vi "Lab Panel V4.90.vi"() -> ()   [LabVIEW 2013] (continued)
                            n2187 = Build Array(w4046) -> (w4034:dbl[])
                            n2188 = Build Array(w4047) -> (w4033:dbl[])
                            n2189 = Build Array(w4042) -> (w4038:dbl[])
                            n2190 = Build Array(w4040) -> (w4037:dbl[])
                            n2191 = Build Array(w4045) -> (w4032:dbl[])
                            n2192 = Build Array("AMPS ON", "AMPS OFF", "VOLTS", "PF", "TEMP Live", "TEMP Neut", "CYCLE") -> (w4015:string[])
                            n2193 = Bundle By Name("Y"=w4038, "t0"=w4031) -> (w4030:waveform(dbl))  [unwired: 1 in]
                            n2194 = Bundle By Name("Y"=w4037, "t0"=w4031) -> (w4029:waveform(dbl))  [unwired: 1 in]
                            n2195 = Bundle By Name("Y"=w4036, "t0"=w4031) -> (w4028:waveform(dbl))  [unwired: 1 in]
                            n2196 = Bundle By Name("Y"=w4035, "t0"=w4031) -> (w4027:waveform(dbl))  [unwired: 1 in]
                            n2197 = Bundle By Name("Y"=w4034, "t0"=w4031) -> (w4026:waveform(dbl))  [unwired: 1 in]
                            n2198 = Bundle By Name("Y"=w4033, "t0"=w4031) -> (w4025:waveform(dbl))  [unwired: 1 in]
                            n2199 = Bundle By Name("Y"=w4032, "t0"=w4031) -> (w4024:waveform(dbl))  [unwired: 1 in]
                            n2200 = Build Array(w4030, w4029, w4028, w4027, w4026, w4025, w4024) -> (w4023:waveform(dbl)[])
                            n2201 = TDMS Write(0:w4044, 5:"TEST VALUES", 7:w4015, 9:w4023) -> (4:w4014:refnum<k34>, 6:w4013:string, 15:w4012:errorcluster)  [unwired: 2 in, 1 out]
                            n2202 = TDMS Write(0:w4014, 5:w4013, 7:"TIME", 9:w4010, 11:w4012) -> (15:w4009:errorcluster)  [unwired: 1 in, 3 out]
                            n2203 = local write "data file error"(w4009) -> ()
                          }
                        }
                      }
                    }
                  }
                }
              }
              frame #4 {
                n2204 = case shown="True" w4048 {
                  tunnel: w4052 -> [_ w4057]
                  tunnel: w4051 -> [_ w4056]
                  tunnel: w4050 -> [_ w4054]
                  tunnel: w4049 -> [_ w4053]
                  frame False {
                  }
                  frame True {
                    n2205 = local read "DISP LAB03-1"() -> (w4058:T4)
                    n2206 = local read "SIG LAB03-1"() -> (w4059:T2)
                    n2207 = local read "ON L03-1"() -> (w4055:cluster{"amps":dbl, "volts":dbl, "pf":dbl})
                    n2208 = Unbundle(w4059) -> ("AMPS"=w4065:dbl, "VOLTS"=w4063:dbl, "PF"=w4062:dbl, "Tmp Live"=w4061:dbl, "Tmp Neut"=w4064:dbl)
                    n2209 = Unbundle(w4058) -> ("CYCLE"=w4060:dbl)  [unwired: 2 out]
                    n2210 = stacked-sequence {
                      tunnel: w4065 -> [w4069 w4088]
                      tunnel: w4064 -> [_ w4087]
                      tunnel: w4063 -> [w4068 w4086]
                      tunnel: w4062 -> [w4067 w4085]
                      tunnel: w4061 -> [_ w4084]
                      tunnel: w4060 -> [_ w4083]
                      tunnel: w4057 -> [_ w4082]
                      tunnel: w4056 -> [w4070 _]
                      tunnel: w4055 -> [w4066 w4080]
                      tunnel: w4054 -> [_ w4081]
                      tunnel: w4053 -> [_ w4076]
                      frame #0 {
                        n2211 = case shown="True" w4070 {
                          tunnel: w4069 -> [_ w4075]
                          tunnel: w4068 -> [_ w4074]
                          tunnel: w4067 -> [_ w4073]
                          tunnel: w4066 -> [_ w4071]
                          frame False {
                          }
                          frame True {
                            n2212 = Bundle(cluster=w4071, "amps"=w4075, "volts"=w4074, "pf"=w4073) -> (w4072:cluster{"amps":dbl, "volts":dbl, "pf":dbl})
                            n2213 = local write "ON L03-1"(w4072) -> ()
                          }
                        }
                      }
                      frame #1 {
                        n2214 = Unbundle(w4080) -> ("amps"=w4079:dbl, "volts"=w4078:dbl, "pf"=w4077:dbl)
                        n2215 = case shown="True" w4081 {
                          tunnel: w4088 -> [_ w4120]
                          tunnel: w4087 -> [_ w4127]
                          tunnel: w4086 -> [_ _]
                          tunnel: w4085 -> [_ _]
                          tunnel: w4084 -> [_ w4126]
                          tunnel: w4083 -> [_ w4125]
                          tunnel: w4082 -> [_ w4090]
                          tunnel: w4079 -> [_ w4122]
                          tunnel: w4078 -> [_ w4121]
                          tunnel: w4077 -> [_ w4119]
                          tunnel: w4076 -> [_ w4111]
                          frame False {
                          }
                          frame True {
                            n2216 = local read "TDMS LAB03-1"() -> (w4124:refnum<k34>)
                            n2217 = Build Array(w4121) -> (w4116:dbl[])
                            n2218 = Build Array(w4119) -> (w4115:dbl[])
                            n2219 = Build Array(w4126) -> (w4114:dbl[])
                            n2220 = Build Array(w4127) -> (w4113:dbl[])
                            n2221 = Build Array(w4122) -> (w4118:dbl[])
                            n2222 = Build Array(w4120) -> (w4117:dbl[])
                            n2223 = Build Array(w4125) -> (w4112:dbl[])
                            n2224 = Build Array("AMPS ON", "AMPS OFF", "VOLTS", "PF", "TEMP Live", "TEMP Neut", "CYCLE") -> (w4095:string[])
                            n2225 = Bundle By Name("Y"=w4118, "t0"=w4111) -> (w4110:waveform(dbl))  [unwired: 1 in]
                            n2226 = Bundle By Name("Y"=w4117, "t0"=w4111) -> (w4109:waveform(dbl))  [unwired: 1 in]
                            n2227 = Bundle By Name("Y"=w4116, "t0"=w4111) -> (w4108:waveform(dbl))  [unwired: 1 in]
                            n2228 = Bundle By Name("Y"=w4115, "t0"=w4111) -> (w4107:waveform(dbl))  [unwired: 1 in]
                            n2229 = Bundle By Name("Y"=w4114, "t0"=w4111) -> (w4106:waveform(dbl))  [unwired: 1 in]
                            n2230 = Bundle By Name("Y"=w4113, "t0"=w4111) -> (w4105:waveform(dbl))  [unwired: 1 in]
                            n2231 = Bundle By Name("Y"=w4112, "t0"=w4111) -> (w4104:waveform(dbl))  [unwired: 1 in]
                            n2232 = Build Array(w4110, w4109, w4108, w4107, w4106, w4105, w4104) -> (w4103:waveform(dbl)[])
                            n2233 = TDMS Write(0:w4124, 5:"TEST VALUES", 7:w4095, 9:w4103) -> (4:w4094:refnum<k34>, 6:w4093:string, 15:w4092:errorcluster)  [unwired: 2 in, 1 out]
                            n2234 = TDMS Write(0:w4094, 5:w4093, 7:"TIME", 9:w4090, 11:w4092) -> (15:w4089:errorcluster)  [unwired: 1 in, 3 out]
                            n2235 = local write "data file error"(w4089) -> ()
                          }
                        }
                      }
                    }
                  }
                }
              }
              frame #5 {
                n2236 = case shown="True" w4128 {
                  tunnel: w4132 -> [_ w4137]
                  tunnel: w4131 -> [_ w4136]
                  tunnel: w4130 -> [_ w4134]
                  tunnel: w4129 -> [_ w4133]
                  frame False {
                  }
                  frame True {
                    n2237 = local read "DISP LAB03-2"() -> (w4138:T4)
                    n2238 = local read "SIG LAB03-2"() -> (w4139:T2)
                    n2239 = local read "ON L03-2"() -> (w4135:cluster{"amps":dbl, "volts":dbl, "pf":dbl})
                    n2240 = Unbundle(w4139) -> ("AMPS"=w4145:dbl, "VOLTS"=w4143:dbl, "PF"=w4142:dbl, "Tmp Live"=w4141:dbl, "Tmp Neut"=w4144:dbl)
                    n2241 = Unbundle(w4138) -> ("CYCLE"=w4140:dbl)  [unwired: 2 out]
                    n2242 = stacked-sequence {
                      tunnel: w4145 -> [w4149 w4168]
                      tunnel: w4144 -> [_ w4167]
                      tunnel: w4143 -> [w4148 w4166]
                      tunnel: w4142 -> [w4147 w4165]
                      tunnel: w4141 -> [_ w4164]
                      tunnel: w4140 -> [_ w4163]
                      tunnel: w4137 -> [_ w4162]
                      tunnel: w4136 -> [w4150 _]
                      tunnel: w4135 -> [w4146 w4160]
                      tunnel: w4134 -> [_ w4161]
                      tunnel: w4133 -> [_ w4156]
                      frame #0 {
                        n2243 = case shown="True" w4150 {
                          tunnel: w4149 -> [_ w4155]
                          tunnel: w4148 -> [_ w4154]
                          tunnel: w4147 -> [_ w4153]
                          tunnel: w4146 -> [_ w4151]
                          frame False {
                          }
                          frame True {
                            n2244 = Bundle(cluster=w4151, "amps"=w4155, "volts"=w4154, "pf"=w4153) -> (w4152:cluster{"amps":dbl, "volts":dbl, "pf":dbl})
                            n2245 = local write "ON L03-2"(w4152) -> ()
                          }
                        }
                      }
                      frame #1 {
                        n2246 = Unbundle(w4160) -> ("amps"=w4159:dbl, "volts"=w4158:dbl, "pf"=w4157:dbl)
                        n2247 = case shown="True" w4161 {
                          tunnel: w4168 -> [_ w4200]
                          tunnel: w4167 -> [_ w4207]
                          tunnel: w4166 -> [_ _]
                          tunnel: w4165 -> [_ _]
                          tunnel: w4164 -> [_ w4206]
                          tunnel: w4163 -> [_ w4205]
                          tunnel: w4162 -> [_ w4170]
                          tunnel: w4159 -> [_ w4202]
                          tunnel: w4158 -> [_ w4201]
                          tunnel: w4157 -> [_ w4199]
                          tunnel: w4156 -> [_ w4191]
                          frame False {
                          }
                          frame True {
                            n2248 = local read "TDMS LAB03-2"() -> (w4204:refnum<k34>)
                            n2249 = Build Array(w4201) -> (w4196:dbl[])
                            n2250 = Build Array(w4199) -> (w4195:dbl[])
                            n2251 = Build Array(w4206) -> (w4194:dbl[])
                            n2252 = Build Array(w4207) -> (w4193:dbl[])
                            n2253 = Build Array(w4202) -> (w4198:dbl[])
                            n2254 = Build Array(w4200) -> (w4197:dbl[])
                            n2255 = Build Array(w4205) -> (w4192:dbl[])
                            n2256 = Build Array("AMPS ON", "AMPS OFF", "VOLTS", "PF", "TEMP Live", "TEMP Neut", "CYCLE") -> (w4175:string[])
                            n2257 = Bundle By Name("Y"=w4198, "t0"=w4191) -> (w4190:waveform(dbl))  [unwired: 1 in]
                            n2258 = Bundle By Name("Y"=w4197, "t0"=w4191) -> (w4189:waveform(dbl))  [unwired: 1 in]
                            n2259 = Bundle By Name("Y"=w4196, "t0"=w4191) -> (w4188:waveform(dbl))  [unwired: 1 in]
                            n2260 = Bundle By Name("Y"=w4195, "t0"=w4191) -> (w4187:waveform(dbl))  [unwired: 1 in]
                            n2261 = Bundle By Name("Y"=w4194, "t0"=w4191) -> (w4186:waveform(dbl))  [unwired: 1 in]
                            n2262 = Bundle By Name("Y"=w4193, "t0"=w4191) -> (w4185:waveform(dbl))  [unwired: 1 in]
                            n2263 = Bundle By Name("Y"=w4192, "t0"=w4191) -> (w4184:waveform(dbl))  [unwired: 1 in]
                            n2264 = Build Array(w4190, w4189, w4188, w4187, w4186, w4185, w4184) -> (w4183:waveform(dbl)[])
                            n2265 = TDMS Write(0:w4204, 5:"TEST VALUES", 7:w4175, 9:w4183) -> (4:w4174:refnum<k34>, 6:w4173:string, 15:w4172:errorcluster)  [unwired: 2 in, 1 out]
                            n2266 = TDMS Write(0:w4174, 5:w4173, 7:"TIME", 9:w4170, 11:w4172) -> (15:w4169:errorcluster)  [unwired: 1 in, 3 out]
                            n2267 = local write "data file error"(w4169) -> ()
                          }
                        }
                      }
                    }
                  }
                }
              }
              frame #6 {
                n2268 = case shown="True" w4208 {
                  tunnel: w4212 -> [_ w4217]
                  tunnel: w4211 -> [_ w4216]
                  tunnel: w4210 -> [_ w4214]
                  tunnel: w4209 -> [_ w4213]
                  frame False {
                  }
                  frame True {
                    n2269 = local read "DISP LAB04-1"() -> (w4218:T4)
                    n2270 = local read "SIG LAB04-1"() -> (w4219:T2)
                    n2271 = local read "ON L04-1"() -> (w4215:cluster{"amps":dbl, "volts":dbl, "pf":dbl})
                    n2272 = Unbundle(w4219) -> ("AMPS"=w4225:dbl, "VOLTS"=w4223:dbl, "PF"=w4222:dbl, "Tmp Live"=w4221:dbl, "Tmp Neut"=w4224:dbl)
                    n2273 = Unbundle(w4218) -> ("CYCLE"=w4220:dbl)  [unwired: 2 out]
                    n2274 = stacked-sequence {
                      tunnel: w4225 -> [w4229 w4248]
                      tunnel: w4224 -> [_ w4247]
                      tunnel: w4223 -> [w4228 w4246]
                      tunnel: w4222 -> [w4227 w4245]
                      tunnel: w4221 -> [_ w4244]
                      tunnel: w4220 -> [_ w4243]
                      tunnel: w4217 -> [_ w4242]
                      tunnel: w4216 -> [w4230 _]
                      tunnel: w4215 -> [w4226 w4240]
                      tunnel: w4214 -> [_ w4241]
                      tunnel: w4213 -> [_ w4236]
                      frame #0 {
                        n2275 = case shown="True" w4230 {
                          tunnel: w4229 -> [_ w4235]
                          tunnel: w4228 -> [_ w4234]
                          tunnel: w4227 -> [_ w4233]
                          tunnel: w4226 -> [_ w4231]
                          frame False {
                          }
                          frame True {
                            n2276 = Bundle(cluster=w4231, "amps"=w4235, "volts"=w4234, "pf"=w4233) -> (w4232:cluster{"amps":dbl, "volts":dbl, "pf":dbl})
                            n2277 = local write "ON L04-1"(w4232) -> ()
                          }
                        }
                      }
                      frame #1 {
                        n2278 = Unbundle(w4240) -> ("amps"=w4239:dbl, "volts"=w4238:dbl, "pf"=w4237:dbl)
                        n2279 = case shown="True" w4241 {
                          tunnel: w4248 -> [_ w4280]
                          tunnel: w4247 -> [_ w4287]
                          tunnel: w4246 -> [_ _]
                          tunnel: w4245 -> [_ _]
                          tunnel: w4244 -> [_ w4286]
                          tunnel: w4243 -> [_ w4285]
                          tunnel: w4242 -> [_ w4250]
                          tunnel: w4239 -> [_ w4282]
                          tunnel: w4238 -> [_ w4281]
                          tunnel: w4237 -> [_ w4279]
                          tunnel: w4236 -> [_ w4271]
                          frame False {
                          }
                          frame True {
                            n2280 = local read "TDMS LAB04-1"() -> (w4284:refnum<k34>)
                            n2281 = Build Array(w4281) -> (w4276:dbl[])
                            n2282 = Build Array(w4279) -> (w4275:dbl[])
                            n2283 = Build Array(w4286) -> (w4274:dbl[])
                            n2284 = Build Array(w4287) -> (w4273:dbl[])
                            n2285 = Build Array(w4282) -> (w4278:dbl[])
                            n2286 = Build Array(w4280) -> (w4277:dbl[])
                            n2287 = Build Array(w4285) -> (w4272:dbl[])
                            n2288 = Build Array("AMPS ON", "AMPS OFF", "VOLTS", "PF", "TEMP Live", "TEMP Neut", "CYCLE") -> (w4255:string[])
                            n2289 = Bundle By Name("Y"=w4278, "t0"=w4271) -> (w4270:waveform(dbl))  [unwired: 1 in]
                            n2290 = Bundle By Name("Y"=w4277, "t0"=w4271) -> (w4269:waveform(dbl))  [unwired: 1 in]
                            n2291 = Bundle By Name("Y"=w4276, "t0"=w4271) -> (w4268:waveform(dbl))  [unwired: 1 in]
                            n2292 = Bundle By Name("Y"=w4275, "t0"=w4271) -> (w4267:waveform(dbl))  [unwired: 1 in]
                            n2293 = Bundle By Name("Y"=w4274, "t0"=w4271) -> (w4266:waveform(dbl))  [unwired: 1 in]
                            n2294 = Bundle By Name("Y"=w4273, "t0"=w4271) -> (w4265:waveform(dbl))  [unwired: 1 in]
                            n2295 = Bundle By Name("Y"=w4272, "t0"=w4271) -> (w4264:waveform(dbl))  [unwired: 1 in]
                            n2296 = Build Array(w4270, w4269, w4268, w4267, w4266, w4265, w4264) -> (w4263:waveform(dbl)[])
                            n2297 = TDMS Write(0:w4284, 5:"TEST VALUES", 7:w4255, 9:w4263) -> (4:w4254:refnum<k34>, 6:w4253:string, 15:w4252:errorcluster)  [unwired: 2 in, 1 out]
                            n2298 = TDMS Write(0:w4254, 5:w4253, 7:"TIME", 9:w4250, 11:w4252) -> (15:w4249:errorcluster)  [unwired: 1 in, 3 out]
                            n2299 = local write "data file error"(w4249) -> ()
                          }
                        }
                      }
                    }
                  }
                }
              }
              frame #7 {
                n2300 = case shown="True" w4288 {
                  tunnel: w4292 -> [_ w4297]
                  tunnel: w4291 -> [_ w4296]
                  tunnel: w4290 -> [_ w4294]
                  tunnel: w4289 -> [_ w4293]
                  frame False {
                  }
                  frame True {
                    n2301 = local read "DISP LAB04-2"() -> (w4298:T4)
                    n2302 = local read "SIG LAB04-2"() -> (w4299:T2)
                    n2303 = local read "ON L04-2"() -> (w4295:cluster{"amps":dbl, "volts":dbl, "pf":dbl})
                    n2304 = Unbundle(w4299) -> ("AMPS"=w4305:dbl, "VOLTS"=w4303:dbl, "PF"=w4302:dbl, "Tmp Live"=w4301:dbl, "Tmp Neut"=w4304:dbl)
                    n2305 = Unbundle(w4298) -> ("CYCLE"=w4300:dbl)  [unwired: 2 out]
                    n2306 = stacked-sequence {
                      tunnel: w4305 -> [w4309 w4328]
                      tunnel: w4304 -> [_ w4327]
                      tunnel: w4303 -> [w4308 w4326]
                      tunnel: w4302 -> [w4307 w4325]
                      tunnel: w4301 -> [_ w4324]
                      tunnel: w4300 -> [_ w4323]
                      tunnel: w4297 -> [_ w4322]
                      tunnel: w4296 -> [w4310 _]
                      tunnel: w4295 -> [w4306 w4320]
                      tunnel: w4294 -> [_ w4321]
                      tunnel: w4293 -> [_ w4316]
                      frame #0 {
                        n2307 = case shown="True" w4310 {
                          tunnel: w4309 -> [_ w4315]
                          tunnel: w4308 -> [_ w4314]
                          tunnel: w4307 -> [_ w4313]
                          tunnel: w4306 -> [_ w4311]
                          frame False {
                          }
                          frame True {
                            n2308 = Bundle(cluster=w4311, "amps"=w4315, "volts"=w4314, "pf"=w4313) -> (w4312:cluster{"amps":dbl, "volts":dbl, "pf":dbl})
                            n2309 = local write "ON L04-2"(w4312) -> ()
                          }
                        }
                      }
                      frame #1 {
                        n2310 = Unbundle(w4320) -> ("amps"=w4319:dbl, "volts"=w4318:dbl, "pf"=w4317:dbl)
                        n2311 = case shown="True" w4321 {
                          tunnel: w4328 -> [_ w4360]
                          tunnel: w4327 -> [_ w4367]
                          tunnel: w4326 -> [_ _]
                          tunnel: w4325 -> [_ _]
                          tunnel: w4324 -> [_ w4366]
                          tunnel: w4323 -> [_ w4365]
                          tunnel: w4322 -> [_ w4330]
                          tunnel: w4319 -> [_ w4362]
                          tunnel: w4318 -> [_ w4361]
                          tunnel: w4317 -> [_ w4359]
                          tunnel: w4316 -> [_ w4351]
                          frame False {
                          }
                          frame True {
                            n2312 = local read "TDMS LAB04-2"() -> (w4364:refnum<k34>)
                            n2313 = Build Array(w4361) -> (w4356:dbl[])
                            n2314 = Build Array(w4359) -> (w4355:dbl[])
                            n2315 = Build Array(w4366) -> (w4354:dbl[])
                            n2316 = Build Array(w4367) -> (w4353:dbl[])
                            n2317 = Build Array(w4362) -> (w4358:dbl[])
                            n2318 = Build Array(w4360) -> (w4357:dbl[])
                            n2319 = Build Array(w4365) -> (w4352:dbl[])
                            n2320 = Build Array("AMPS ON", "AMPS OFF", "VOLTS", "PF", "TEMP Live", "TEMP Neut", "CYCLE") -> (w4335:string[])
                            n2321 = Bundle By Name("Y"=w4358, "t0"=w4351) -> (w4350:waveform(dbl))  [unwired: 1 in]
                            n2322 = Bundle By Name("Y"=w4357, "t0"=w4351) -> (w4349:waveform(dbl))  [unwired: 1 in]
                            n2323 = Bundle By Name("Y"=w4356, "t0"=w4351) -> (w4348:waveform(dbl))  [unwired: 1 in]
                            n2324 = Bundle By Name("Y"=w4355, "t0"=w4351) -> (w4347:waveform(dbl))  [unwired: 1 in]
                            n2325 = Bundle By Name("Y"=w4354, "t0"=w4351) -> (w4346:waveform(dbl))  [unwired: 1 in]
                            n2326 = Bundle By Name("Y"=w4353, "t0"=w4351) -> (w4345:waveform(dbl))  [unwired: 1 in]
                            n2327 = Bundle By Name("Y"=w4352, "t0"=w4351) -> (w4344:waveform(dbl))  [unwired: 1 in]
                            n2328 = Build Array(w4350, w4349, w4348, w4347, w4346, w4345, w4344) -> (w4343:waveform(dbl)[])
                            n2329 = TDMS Write(0:w4364, 5:"TEST VALUES", 7:w4335, 9:w4343) -> (4:w4334:refnum<k34>, 6:w4333:string, 15:w4332:errorcluster)  [unwired: 2 in, 1 out]
                            n2330 = TDMS Write(0:w4334, 5:w4333, 7:"TIME", 9:w4330, 11:w4332) -> (15:w4329:errorcluster)  [unwired: 1 in, 3 out]
                            n2331 = local write "data file error"(w4329) -> ()
                          }
                        }
                      }
                    }
                  }
                }
              }
              frame #8 {
                n2332 = case shown="True" w4368 {
                  tunnel: w4372 -> [_ w4377]
                  tunnel: w4371 -> [_ w4376]
                  tunnel: w4370 -> [_ w4374]
                  tunnel: w4369 -> [_ w4373]
                  frame False {
                  }
                  frame True {
                    n2333 = local read "DISP LAB05-1"() -> (w4378:T4)
                    n2334 = local read "SIG LAB05-1"() -> (w4379:T2)
                    n2335 = local read "ON L05-1"() -> (w4375:cluster{"amps":dbl, "volts":dbl, "pf":dbl})
                    n2336 = Unbundle(w4379) -> ("AMPS"=w4385:dbl, "VOLTS"=w4383:dbl, "PF"=w4382:dbl, "Tmp Live"=w4381:dbl, "Tmp Neut"=w4384:dbl)
                    n2337 = Unbundle(w4378) -> ("CYCLE"=w4380:dbl)  [unwired: 2 out]
                    n2338 = stacked-sequence {
                      tunnel: w4385 -> [w4389 w4408]
                      tunnel: w4384 -> [_ w4407]
                      tunnel: w4383 -> [w4388 w4406]
                      tunnel: w4382 -> [w4387 w4405]
                      tunnel: w4381 -> [_ w4404]
                      tunnel: w4380 -> [_ w4403]
                      tunnel: w4377 -> [_ w4402]
                      tunnel: w4376 -> [w4390 _]
                      tunnel: w4375 -> [w4386 w4400]
                      tunnel: w4374 -> [_ w4401]
                      tunnel: w4373 -> [_ w4396]
                      frame #0 {
                        n2339 = case shown="True" w4390 {
                          tunnel: w4389 -> [_ w4395]
                          tunnel: w4388 -> [_ w4394]
                          tunnel: w4387 -> [_ w4393]
                          tunnel: w4386 -> [_ w4391]
                          frame False {
                          }
                          frame True {
                            n2340 = Bundle(cluster=w4391, "amps"=w4395, "volts"=w4394, "pf"=w4393) -> (w4392:cluster{"amps":dbl, "volts":dbl, "pf":dbl})
                            n2341 = local write "ON L05-1"(w4392) -> ()
                          }
                        }
                      }
                      frame #1 {
                        n2342 = Unbundle(w4400) -> ("amps"=w4399:dbl, "volts"=w4398:dbl, "pf"=w4397:dbl)
                        n2343 = case shown="True" w4401 {
                          tunnel: w4408 -> [_ w4440]
                          tunnel: w4407 -> [_ w4447]
                          tunnel: w4406 -> [_ _]
                          tunnel: w4405 -> [_ _]
                          tunnel: w4404 -> [_ w4446]
                          tunnel: w4403 -> [_ w4445]
                          tunnel: w4402 -> [_ w4410]
                          tunnel: w4399 -> [_ w4442]
                          tunnel: w4398 -> [_ w4441]
                          tunnel: w4397 -> [_ w4439]
                          tunnel: w4396 -> [_ w4431]
                          frame False {
                          }
                          frame True {
                            n2344 = local read "TDMS LAB05-1"() -> (w4444:refnum<k34>)
                            n2345 = Build Array(w4441) -> (w4436:dbl[])
                            n2346 = Build Array(w4439) -> (w4435:dbl[])
                            n2347 = Build Array(w4446) -> (w4434:dbl[])
                            n2348 = Build Array(w4447) -> (w4433:dbl[])
                            n2349 = Build Array(w4442) -> (w4438:dbl[])
                            n2350 = Build Array(w4440) -> (w4437:dbl[])
                            n2351 = Build Array(w4445) -> (w4432:dbl[])
                            n2352 = Build Array("AMPS ON", "AMPS OFF", "VOLTS", "PF", "TEMP Live", "TEMP Neut", "CYCLE") -> (w4415:string[])
                            n2353 = Bundle By Name("Y"=w4438, "t0"=w4431) -> (w4430:waveform(dbl))  [unwired: 1 in]
                            n2354 = Bundle By Name("Y"=w4437, "t0"=w4431) -> (w4429:waveform(dbl))  [unwired: 1 in]
                            n2355 = Bundle By Name("Y"=w4436, "t0"=w4431) -> (w4428:waveform(dbl))  [unwired: 1 in]
                            n2356 = Bundle By Name("Y"=w4435, "t0"=w4431) -> (w4427:waveform(dbl))  [unwired: 1 in]
                            n2357 = Bundle By Name("Y"=w4434, "t0"=w4431) -> (w4426:waveform(dbl))  [unwired: 1 in]
                            n2358 = Bundle By Name("Y"=w4433, "t0"=w4431) -> (w4425:waveform(dbl))  [unwired: 1 in]
                            n2359 = Bundle By Name("Y"=w4432, "t0"=w4431) -> (w4424:waveform(dbl))  [unwired: 1 in]
                            n2360 = Build Array(w4430, w4429, w4428, w4427, w4426, w4425, w4424) -> (w4423:waveform(dbl)[])
                            n2361 = TDMS Write(0:w4444, 5:"TEST VALUES", 7:w4415, 9:w4423) -> (4:w4414:refnum<k34>, 6:w4413:string, 15:w4412:errorcluster)  [unwired: 2 in, 1 out]
                            n2362 = TDMS Write(0:w4414, 5:w4413, 7:"TIME", 9:w4410, 11:w4412) -> (15:w4409:errorcluster)  [unwired: 1 in, 3 out]
                            n2363 = local write "data file error"(w4409) -> ()
                          }
                        }
                      }
                    }
                  }
                }
              }
              frame #9 {
                n2364 = case shown="True" w4448 {
                  tunnel: w4452 -> [_ w4457]
                  tunnel: w4451 -> [_ w4456]
                  tunnel: w4450 -> [_ w4454]
                  tunnel: w4449 -> [_ w4453]
                  frame False {
                  }
                  frame True {
                    n2365 = local read "DISP LAB05-2"() -> (w4458:T4)
                    n2366 = local read "SIG LAB05-2"() -> (w4459:T2)
                    n2367 = local read "ON L05-2"() -> (w4455:cluster{"amps":dbl, "volts":dbl, "pf":dbl})
                    n2368 = Unbundle(w4459) -> ("AMPS"=w4465:dbl, "VOLTS"=w4463:dbl, "PF"=w4462:dbl, "Tmp Live"=w4461:dbl, "Tmp Neut"=w4464:dbl)
                    n2369 = Unbundle(w4458) -> ("CYCLE"=w4460:dbl)  [unwired: 2 out]
                    n2370 = stacked-sequence {
                      tunnel: w4465 -> [w4469 w4488]
                      tunnel: w4464 -> [_ w4487]
                      tunnel: w4463 -> [w4468 w4486]
                      tunnel: w4462 -> [w4467 w4485]
                      tunnel: w4461 -> [_ w4484]
                      tunnel: w4460 -> [_ w4483]
                      tunnel: w4457 -> [_ w4482]
                      tunnel: w4456 -> [w4470 _]
                      tunnel: w4455 -> [w4466 w4480]
                      tunnel: w4454 -> [_ w4481]
                      tunnel: w4453 -> [_ w4476]
                      frame #0 {
                        n2371 = case shown="True" w4470 {
                          tunnel: w4469 -> [_ w4475]
                          tunnel: w4468 -> [_ w4474]
                          tunnel: w4467 -> [_ w4473]
                          tunnel: w4466 -> [_ w4471]
                          frame False {
                          }
                          frame True {
                            n2372 = Bundle(cluster=w4471, "amps"=w4475, "volts"=w4474, "pf"=w4473) -> (w4472:cluster{"amps":dbl, "volts":dbl, "pf":dbl})
                            n2373 = local write "ON L05-2"(w4472) -> ()
                          }
                        }
                      }
                      frame #1 {
                        n2374 = Unbundle(w4480) -> ("amps"=w4479:dbl, "volts"=w4478:dbl, "pf"=w4477:dbl)
                        n2375 = case shown="True" w4481 {
                          tunnel: w4488 -> [_ w4520]
                          tunnel: w4487 -> [_ w4527]
                          tunnel: w4486 -> [_ _]
                          tunnel: w4485 -> [_ _]
                          tunnel: w4484 -> [_ w4526]
                          tunnel: w4483 -> [_ w4525]
                          tunnel: w4482 -> [_ w4490]
                          tunnel: w4479 -> [_ w4522]
                          tunnel: w4478 -> [_ w4521]
                          tunnel: w4477 -> [_ w4519]
                          tunnel: w4476 -> [_ w4511]
                          frame False {
                          }
                          frame True {
                            n2376 = local read "TDMS LAB05-2"() -> (w4524:refnum<k34>)
                            n2377 = Build Array(w4521) -> (w4516:dbl[])
                            n2378 = Build Array(w4519) -> (w4515:dbl[])
                            n2379 = Build Array(w4526) -> (w4514:dbl[])
                            n2380 = Build Array(w4527) -> (w4513:dbl[])
                            n2381 = Build Array(w4522) -> (w4518:dbl[])
                            n2382 = Build Array(w4520) -> (w4517:dbl[])
                            n2383 = Build Array(w4525) -> (w4512:dbl[])
                            n2384 = Build Array("AMPS ON", "AMPS OFF", "VOLTS", "PF", "TEMP Live", "TEMP Neut", "CYCLE") -> (w4495:string[])
                            n2385 = Bundle By Name("Y"=w4518, "t0"=w4511) -> (w4510:waveform(dbl))  [unwired: 1 in]
                            n2386 = Bundle By Name("Y"=w4517, "t0"=w4511) -> (w4509:waveform(dbl))  [unwired: 1 in]
                            n2387 = Bundle By Name("Y"=w4516, "t0"=w4511) -> (w4508:waveform(dbl))  [unwired: 1 in]
                            n2388 = Bundle By Name("Y"=w4515, "t0"=w4511) -> (w4507:waveform(dbl))  [unwired: 1 in]
                            n2389 = Bundle By Name("Y"=w4514, "t0"=w4511) -> (w4506:waveform(dbl))  [unwired: 1 in]
                            n2390 = Bundle By Name("Y"=w4513, "t0"=w4511) -> (w4505:waveform(dbl))  [unwired: 1 in]
                            n2391 = Bundle By Name("Y"=w4512, "t0"=w4511) -> (w4504:waveform(dbl))  [unwired: 1 in]
                            n2392 = Build Array(w4510, w4509, w4508, w4507, w4506, w4505, w4504) -> (w4503:waveform(dbl)[])
                            n2393 = TDMS Write(0:w4524, 5:"TEST VALUES", 7:w4495, 9:w4503) -> (4:w4494:refnum<k34>, 6:w4493:string, 15:w4492:errorcluster)  [unwired: 2 in, 1 out]
                            n2394 = TDMS Write(0:w4494, 5:w4493, 7:"TIME", 9:w4490, 11:w4492) -> (15:w4489:errorcluster)  [unwired: 1 in, 3 out]
                            n2395 = local write "data file error"(w4489) -> ()
                          }
                        }
                      }
                    }
                  }
                }
              }
            }
          }
          frame #13 {
            # "display test values on chart"
            n2396 = local read "jig cycle"() -> (w4532:dbl)
            n2397 = local read "on loops"() -> (w4534:dbl)
            n2398 = Add(x=w4534, y=2) -> (x+y=w4531:dbl)
            n2399 = Equal?(x=w4532, y=1) -> (x = y?=w4530:bool)
            n2400 = Equal?(x=w4532, y=w4531) -> (x = y?=w4529:bool)
            n2401 = Or(x=w4530, y=w4529) -> (x .or. y?=w4528:bool)
            "graph flag" <- w4528
            n2402 = global write "Global display 3.vi" "graph flag"(w4528) -> ()
            n2403 = case shown="True" w4528 {
              frame False {
              }
              frame True {
                n2404 = local read "SIG LAB05-1"() -> (w4577:T2)
                n2405 = local read "SIG LAB04-2"() -> (w4578:T2)
                n2406 = local read "SIG LAB05-2"() -> (w4576:T2)
                n2407 = local read "SIG LAB04-1"() -> (w4579:T2)
                n2408 = local read "SIG LAB03-1"() -> (w4581:T2)
                n2409 = local read "SIG LAB03-2"() -> (w4580:T2)
                n2410 = local read "SIG LAB01-1"() -> (w4585:T2)
                n2411 = local read "SIG LAB02-2"() -> (w4582:T2)
                n2412 = local read "SIG LAB02-1"() -> (w4583:T2)
                n2413 = local read "SIG LAB01-2"() -> (w4584:T2)
                n2414 = Unbundle(w4578) -> ("AMPS"=w4568:dbl, "VOLTS"=w4558:dbl, "Tmp Live"=w4548:dbl, "Tmp Neut"=w4538:dbl)  [unwired: 1 out]
                n2415 = Unbundle(w4577) -> ("AMPS"=w4567:dbl, "VOLTS"=w4557:dbl, "Tmp Live"=w4547:dbl, "Tmp Neut"=w4537:dbl)  [unwired: 1 out]
                n2416 = Unbundle(w4576) -> ("AMPS"=w4566:dbl, "VOLTS"=w4556:dbl, "Tmp Live"=w4546:dbl, "Tmp Neut"=w4536:dbl)  [unwired: 1 out]
                n2417 = Unbundle(w4579) -> ("AMPS"=w4569:dbl, "VOLTS"=w4559:dbl, "Tmp Live"=w4549:dbl, "Tmp Neut"=w4539:dbl)  [unwired: 1 out]
                n2418 = Unbundle(w4580) -> ("AMPS"=w4570:dbl, "VOLTS"=w4560:dbl, "Tmp Live"=w4550:dbl, "Tmp Neut"=w4540:dbl)  [unwired: 1 out]
                n2419 = Unbundle(w4581) -> ("AMPS"=w4571:dbl, "VOLTS"=w4561:dbl, "Tmp Live"=w4551:dbl, "Tmp Neut"=w4541:dbl)  [unwired: 1 out]
                n2420 = Unbundle(w4582) -> ("AMPS"=w4572:dbl, "VOLTS"=w4562:dbl, "Tmp Live"=w4552:dbl, "Tmp Neut"=w4542:dbl)  [unwired: 1 out]
                n2421 = Unbundle(w4583) -> ("AMPS"=w4573:dbl, "VOLTS"=w4563:dbl, "Tmp Live"=w4553:dbl, "Tmp Neut"=w4543:dbl)  [unwired: 1 out]
                n2422 = Unbundle(w4585) -> ("AMPS"=w4575:dbl, "VOLTS"=w4565:dbl, "Tmp Live"=w4555:dbl, "Tmp Neut"=w4545:dbl)  [unwired: 1 out]
                n2423 = Unbundle(w4584) -> ("AMPS"=w4574:dbl, "VOLTS"=w4564:dbl, "Tmp Live"=w4554:dbl, "Tmp Neut"=w4544:dbl)  [unwired: 1 out]
                n2424 = stacked-sequence {
                  tunnel: w4575 -> [w4617 _ _]
                  tunnel: w4574 -> [w4616 _ _]
                  tunnel: w4573 -> [w4607 _ _]
                  tunnel: w4572 -> [w4606 _ _]
                  tunnel: w4571 -> [w4596 _ _]
                  tunnel: w4570 -> [w4595 _ _]
                  tunnel: w4569 -> [_ w4640 _]
                  tunnel: w4568 -> [_ w4639 _]
                  tunnel: w4567 -> [_ w4629 _]
                  tunnel: w4566 -> [_ w4628 _]
                  tunnel: w4565 -> [w4614 _ _]
                  tunnel: w4564 -> [w4613 _ _]
                  tunnel: w4563 -> [w4604 _ _]
                  tunnel: w4562 -> [w4603 _ _]
                  tunnel: w4561 -> [w4594 _ _]
                  tunnel: w4560 -> [w4593 _ _]
                  tunnel: w4559 -> [_ w4638 _]
                  tunnel: w4558 -> [_ w4637 _]
                  tunnel: w4557 -> [_ w4627 _]
                  tunnel: w4556 -> [_ w4626 _]
                  tunnel: w4555 -> [w4611 _ _]
                  tunnel: w4554 -> [w4609 _ _]
                  tunnel: w4553 -> [w4600 _ _]
                  tunnel: w4552 -> [w4598 _ _]
                  tunnel: w4551 -> [w4592 _ _]
                  tunnel: w4550 -> [w4590 _ _]
                  tunnel: w4549 -> [_ w4636 _]
                  tunnel: w4548 -> [_ w4634 _]
                  tunnel: w4547 -> [_ w4625 _]
                  tunnel: w4546 -> [_ w4623 _]
                  tunnel: w4545 -> [w4610 _ _]
                  tunnel: w4544 -> [w4608 _ _]
                  tunnel: w4543 -> [w4599 _ _]
                  tunnel: w4542 -> [w4597 _ _]
                  tunnel: w4541 -> [w4591 _ _]
                  tunnel: w4540 -> [w4589 _ _]
                  tunnel: w4539 -> [_ w4635 _]
                  tunnel: w4538 -> [_ w4633 _]
                  tunnel: w4537 -> [_ w4624 _]
                  tunnel: w4536 -> [_ w4622 _]
                  frame #0 {
                    n2425 = Merge Signals(w4617, w4616) -> (→"LAB01 AMPS":dynamicdata)
                    n2426 = Merge Signals(w4614, w4613) -> (→"LAB01 VOLTS":dynamicdata)
                    n2427 = Merge Signals(w4594, w4593) -> (→"LAB03 VOLTS":dynamicdata)
                    n2428 = Merge Signals(w4611, w4610, w4609, w4608) -> (→"LAB01 deg C":dynamicdata)
                    n2429 = Merge Signals(w4607, w4606) -> (→"LAB02 AMPS":dynamicdata)
                    n2430 = Merge Signals(w4600, w4599, w4598, w4597) -> (→"LAB02 deg C":dynamicdata)
                    n2431 = Merge Signals(w4592, w4591, w4590, w4589) -> (→"LAB03 deg C":dynamicdata)
                    n2432 = Merge Signals(w4604, w4603) -> (→"LAB02 VOLTS":dynamicdata)
                    n2433 = Merge Signals(w4596, w4595) -> (→"LAB03 AMPS":dynamicdata)
                  }
                  frame #1 {
                    n2434 = Merge Signals(w4627, w4626) -> (→"LAB05 VOLTS":dynamicdata)
                    n2435 = Merge Signals(w4640, w4639) -> (→"LAB04 AMPS":dynamicdata)
                    n2436 = Merge Signals(w4629, w4628) -> (→"LAB05 AMPS":dynamicdata)
                    n2437 = Merge Signals(w4625, w4624, w4623, w4622) -> (→"LAB05 deg C":dynamicdata)
                    n2438 = Merge Signals(w4636, w4635, w4634, w4633) -> (→"LAB04 deg C":dynamicdata)
                    n2439 = Merge Signals(w4638, w4637) -> (→"LAB04 VOLTS":dynamicdata)
                  }
                  frame #2 {
                    n2440 = local read "LAB05 VOLTS"() -> (w4648:dynamicdata)
                    n2441 = local read "LAB04 VOLTS"() -> (w4649:dynamicdata)
                    n2442 = local read "LAB02 VOLTS"() -> (w4651:dynamicdata)
                    n2443 = local read "LAB03 VOLTS"() -> (w4650:dynamicdata)
                    n2444 = local read "LAB05 AMPS"() -> (w4654:dynamicdata)
                    n2445 = local read "LAB01 VOLTS"() -> (w4652:dynamicdata)
                    n2446 = local read "LAB04 AMPS"() -> (w4655:dynamicdata)
                    n2447 = local read "LAB03 AMPS"() -> (w4656:dynamicdata)
                    n2448 = local read "LAB03 deg C"() -> (w4644:dynamicdata)
                    n2449 = local read "LAB02 AMPS"() -> (w4657:dynamicdata)
                    n2450 = local read "LAB04 deg C"() -> (w4643:dynamicdata)
                    n2451 = local read "LAB05 deg C"() -> (w4642:dynamicdata)
                    n2452 = local read "LAB02 deg C"() -> (w4645:dynamicdata)
                    n2453 = local read "LAB01 deg C"() -> (w4646:dynamicdata)
                    n2454 = local read "LAB01 AMPS"() -> (w4658:dynamicdata)
                    n2455 = Merge Signals(w4646, w4645, w4644, w4643, w4642) -> (w4641:dynamicdata)
                    n2456 = Merge Signals(w4658, w4657, w4656, w4655, w4654) -> (w4653:dynamicdata)
                    n2457 = Merge Signals(w4652, w4651, w4650, w4649, w4648) -> (w4647:dynamicdata)
                    n2458 = global write "Global display 3.vi" "graph volts"(w4647) -> ()
                    n2459 = global write "Global display 3.vi" "graph deg C"(w4641) -> ()
                    n2460 = global write "Global display 3.vi" "graph amps"(w4653) -> ()
                  }
                }
              }
            }
          }
          frame #14 {
            # "check for amps fail"
            # "check for cycle test & temperature rise fail conditions"
            n2461 = local read "on loops"() -> (w4685:dbl)
            n2462 = local read "jig cycle"() -> (w4682:dbl)
            n2463 = local read "jig cycle"() -> (w4687:dbl)
            n2464 = Add(x=w4685, y=3.0) -> (x+y=w4683:dbl)
            n2465 = Equal?(x=w4682, y=w4683) -> (x = y?=w4678:bool)
            n2466 = local read "Fail Loops"() -> (w4659:dbl)
            n2467 = Equal?(x=w4687, y=1.0) -> (x = y?=w4680:bool)
            n2468 = global write "Global 1.vi" "fail count"(w4659) -> ()
            n2469 = stacked-sequence {
              tunnel: w4681 -> [w4690 _ _ _ _ _ _ _ _ _]
              tunnel: w4680 -> [w4691 w4711 w4731 w4751 w4771 w4791 w4811 w4831 w4851 w4871]
              tunnel: w4679 -> [w4688 _ _ _ _ _ _ _ _ _]
              tunnel: w4678 -> [w4689 w4710 w4730 w4750 w4770 w4790 w4810 w4830 w4850 w4870]
              tunnel: w4677 -> [_ w4709 _ _ _ _ _ _ _ _]
              tunnel: w4676 -> [_ w4708 _ _ _ _ _ _ _ _]
              tunnel: w4675 -> [_ _ w4729 _ _ _ _ _ _ _]
              tunnel: w4674 -> [_ _ w4728 _ _ _ _ _ _ _]
              tunnel: w4673 -> [_ _ _ w4749 _ _ _ _ _ _]
              tunnel: w4672 -> [_ _ _ w4748 _ _ _ _ _ _]
              tunnel: w4671 -> [_ _ _ _ w4769 _ _ _ _ _]
              tunnel: w4670 -> [_ _ _ _ w4768 _ _ _ _ _]
              tunnel: w4669 -> [_ _ _ _ _ w4789 _ _ _ _]
              tunnel: w4668 -> [_ _ _ _ _ w4788 _ _ _ _]
              tunnel: w4667 -> [_ _ _ _ _ _ w4809 _ _ _]
              tunnel: w4666 -> [_ _ _ _ _ _ w4808 _ _ _]
              tunnel: w4665 -> [_ _ _ _ _ _ _ w4829 _ _]
              tunnel: w4664 -> [_ _ _ _ _ _ _ w4828 _ _]
              tunnel: w4663 -> [_ _ _ _ _ _ _ _ w4849 _]
              tunnel: w4662 -> [_ _ _ _ _ _ _ _ w4848 _]
              tunnel: w4661 -> [_ _ _ _ _ _ _ _ _ w4869]
              tunnel: w4660 -> [_ _ _ _ _ _ _ _ _ w4868]
              frame #0 {
                # "LAB01-1"
                n2470 = case shown="True" w4688 {
                  tunnel: w4691 -> [_ w4704]
                  tunnel: w4690 -> [_ w4701]
                  tunnel: w4689 -> [_ w4700]
                  frame False {
                  }
                  frame True {
                    n2471 = local read "TEMP START LAB01-1"() -> (w4706:cluster{"TL":dbl, "TN":dbl})
                    n2472 = local read "RESULT LAB01-1"() -> (w4695:bool)
                    n2473 = local read "FAIL LAB01-1"() -> (w4698:cluster{"LO":dbl, "HI":dbl})
                    n2474 = local read "TDMS LAB01-1"() -> (w4705:refnum<k34>)
                    n2475 = local read "SET LAB01-1"() -> (w4702:T5)
                    n2476 = local read "DISP LAB01-1"() -> (w4703:T4)
                    n2477 = local read "SIG LAB01-1"() -> (w4707:T2)
                    n2478 = Bundle("FAIL LAB01-1"=w4698, "SIG LAB01-1"=w4707, "TEMP START LAB01-1"=w4706, "DISP LAB01-1"=w4703, "SET LAB01-1"=w4702, "TDMS LAB01-1"=w4705) -> (w4692:T32)  [unwired: 1 in]
                    n2479 = call "sub vi - cycle&temp fail v7.vi"("Amps Lo?"=w4704, "Input Cluster"=w4692, "SELECT"=w4701, "Amps Hi?"=w4700, "Result In"=w4695) -> ("(FAIL) out"=w4697:cluster{"FAIL LO":dbl, "FAIL HI":dbl}, "(DISP) out"=w4693:T4, "T-RISE"=w4694:cluster{"T-RISE (L)":dbl, "T-RISE (N)":dbl}, "Result Out"=w4696:bool, "file error"=w4699:errorcluster)  [unwired: 10 in]
                    n2480 = local write "TEMP RISE LAB01-1"(w4694) -> ()
                    n2481 = local write "FAIL LAB01-1"(w4697) -> ()
                    n2482 = local write "DISP LAB01-1"(w4693) -> ()
                    n2483 = local write "RESULT LAB01-1"(w4696) -> ()
                    n2484 = local write "data file error"(w4699) -> ()
                  }
                }
              }
              frame #1 {
                # "LAB01-2"
                n2485 = case shown="True" w4709 {
                  tunnel: w4711 -> [_ w4724]
                  tunnel: w4708 -> [_ w4721]
                  tunnel: w4710 -> [_ w4720]
                  frame False {
                  }
                  frame True {
                    n2486 = local read "TEMP START LAB01-2"() -> (w4726:cluster{"TL":dbl, "TN":dbl})
                    n2487 = local read "FAIL LAB01-2"() -> (w4717:cluster{"LO":dbl, "HI":dbl})
                    n2488 = local read "TDMS LAB01-2"() -> (w4725:refnum<k34>)
                    n2489 = local read "SET LAB01-2"() -> (w4722:T5)
                    n2490 = local read "DISP LAB01-2"() -> (w4723:T4)
                    n2491 = local read "RESULT LAB01-2"() -> (w4714:bool)
                    n2492 = local read "SIG LAB01-2"() -> (w4727:T2)
                    n2493 = Bundle("FAIL LAB01-2"=w4717, "SIG LAB01-2"=w4727, "TEMP START LAB01-2"=w4726, "DISP LAB01-2"=w4723, "SET LAB01-2"=w4722, "TDMS LAB01-2"=w4725) -> (w4712:T33)  [unwired: 1 in]
                    n2494 = call "sub vi - cycle&temp fail v7.vi"("Amps Lo?"=w4724, "Input Cluster"=w4712, "SELECT"=w4721, "Amps Hi?"=w4720, "Result In"=w4714) -> ("(FAIL) out"=w4716:cluster{"FAIL LO":dbl, "FAIL HI":dbl}, "(DISP) out"=w4719:T4, "T-RISE"=w4713:cluster{"T-RISE (L)":dbl, "T-RISE (N)":dbl}, "Result Out"=w4715:bool, "file error"=w4718:errorcluster)  [unwired: 10 in]
                    n2495 = local write "TEMP RISE LAB01-2"(w4713) -> ()
                    n2496 = local write "FAIL LAB01-2"(w4716) -> ()
                    n2497 = local write "DISP LAB01-2"(w4719) -> ()
                    n2498 = local write "RESULT LAB01-2"(w4715) -> ()
                    n2499 = local write "data file error"(w4718) -> ()
                  }
                }
              }
              frame #2 {
                # "LAB02-1"
                n2500 = case shown="True" w4729 {
                  tunnel: w4731 -> [_ w4744]
                  tunnel: w4728 -> [_ w4741]
                  tunnel: w4730 -> [_ w4740]
                  frame False {
                  }
                  frame True {
                    n2501 = local read "TEMP START LAB02-1"() -> (w4746:cluster{"TL":dbl, "TN":dbl})
                    n2502 = local read "FAIL LAB02-1"() -> (w4737:cluster{"LO":dbl, "HI":dbl})
                    n2503 = local read "TDMS LAB02-1"() -> (w4745:refnum<k34>)
                    n2504 = local read "SET LAB02-1"() -> (w4742:T5)
                    n2505 = local read "DISP LAB02-1"() -> (w4743:T4)
                    n2506 = local read "SIG LAB02-1"() -> (w4747:T2)
                    n2507 = local read "RESULT LAB02-1"() -> (w4734:bool)
                    n2508 = Bundle("FAIL LAB02-1"=w4737, "SIG LAB02-1"=w4747, "TEMP START LAB02-1"=w4746, "DISP LAB02-1"=w4743, "SET LAB02-1"=w4742, "TDMS LAB02-1"=w4745) -> (w4732:T34)  [unwired: 1 in]
                    n2509 = call "sub vi - cycle&temp fail v7.vi"("Amps Lo?"=w4744, "Input Cluster"=w4732, "SELECT"=w4741, "Amps Hi?"=w4740, "Result In"=w4734) -> ("(FAIL) out"=w4736:cluster{"FAIL LO":dbl, "FAIL HI":dbl}, "(DISP) out"=w4739:T4, "T-RISE"=w4733:cluster{"T-RISE (L)":dbl, "T-RISE (N)":dbl}, "Result Out"=w4735:bool, "file error"=w4738:errorcluster)  [unwired: 10 in]
                    n2510 = local write "TEMP RISE LAB02-1"(w4733) -> ()
                    n2511 = local write "FAIL LAB02-1"(w4736) -> ()
                    n2512 = local write "DISP LAB02-1"(w4739) -> ()
                    n2513 = local write "RESULT LAB02-1"(w4735) -> ()
                    n2514 = local write "data file error"(w4738) -> ()
                  }
                }
              }
              frame #3 {
                # "LAB02-2"
                n2515 = case shown="True" w4749 {
                  tunnel: w4751 -> [_ w4764]
                  tunnel: w4748 -> [_ w4761]
                  tunnel: w4750 -> [_ w4760]
                  frame False {
                  }
                  frame True {
                    n2516 = local read "TEMP START LAB02-2"() -> (w4766:cluster{"TL":dbl, "TN":dbl})
                    n2517 = local read "FAIL LAB02-2"() -> (w4757:cluster{"LO":dbl, "HI":dbl})
                    n2518 = local read "TDMS LAB02-2"() -> (w4765:refnum<k34>)
                    n2519 = local read "SET LAB02-2"() -> (w4762:T5)
                    n2520 = local read "DISP LAB02-2"() -> (w4763:T4)
